vi "atMonochromator_getEvent_settingsAppliedLoop.vi"(8 "error in (no error)":errorcluster, 11 "logevent_settingsAppliedLoop_Ctl":T1) -> (0 "error out":errorcluster, 2 "function return":i32, 3 "logevent_settingsAppliedLoop_Ctl out":T1)   [LabVIEW 2016, in "SALLV_atMonochromator.lvlib"]
doc: "int atMonochromator_shm_getEvent_settingsAppliedLoopLV(atMonochromator_logevent_settingsAppliedLoopLV *logevent_settingsAppliedLoop_Ctl );"
uses:
  SALLV_atMonochromator.lvlib
  DataTypes/logevent_settingsAppliedLoop.ctl
  SALLV_atMonochromator.so
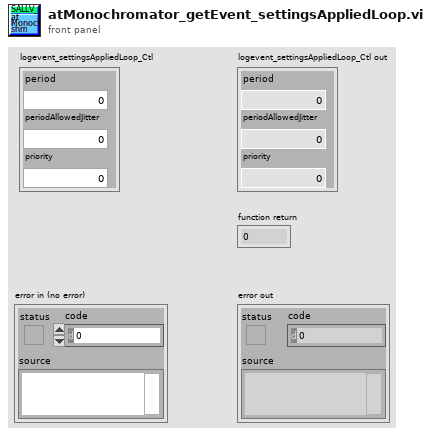
[diagram p1: front panel]
types:
  T1 = typedef "SALLV_atMonochromator.lvlib/logevent_settingsAppliedLoop.ctl" = cluster{"period":dbl, "periodAllowedJitter":dbl, "priority":i32}
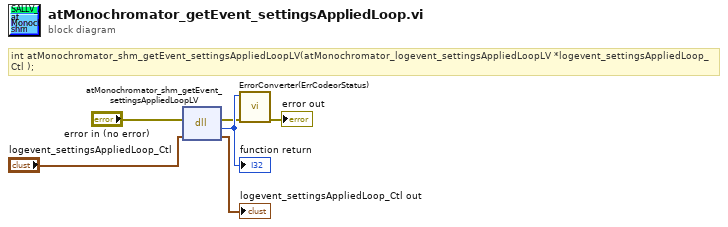
[diagram p0: block diagram]
diagram:
  # "int atMonochromator_shm_getEvent_settingsAppliedLoopLV(atMonochromator_logevent_settingsAppliedLoopLV *logevent_settingsAppliedLoop_Ctl );"
  n1 = dll-call lib="home/andres/Desktop/SAL_atMonochromator/SALLV_atMonochromator.*" fn="atMonochromator_shm_getEvent_settingsAppliedLoopLV"(error in="error in (no error)", "logevent_settingsAppliedLoop_Ctl"="logevent_settingsAppliedLoop_Ctl") -> (error out=w2:errorcluster, w6:i32, "logevent_settingsAppliedLoop_Ctl"=→"logevent_settingsAppliedLoop_Ctl out":T1)  [unwired: 2 in, 1 out]
  "function return" <- w6
  n2 = call "ErrorConverter(ErrCodeorStatus).vi"("error in (no error)"=w2, "error code"=w6) -> ("error out"=→"error out":errorcluster)  [unwired: 9 in]
